vi "ITU_Amplitude(Frequency Domain).vi"(9 "Frequency":dbl=1000.0 format="%#_13g", 10 "Amplitude":dbl=1.0 format="%#_13g") -> (1 "Amplitude_output":dbl)   [LabVIEW 2015]
doc: "Use this VI to calculate ITU-468 filtered amplitude of a signals FFT"
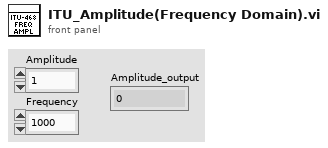
[diagram p1: front panel]
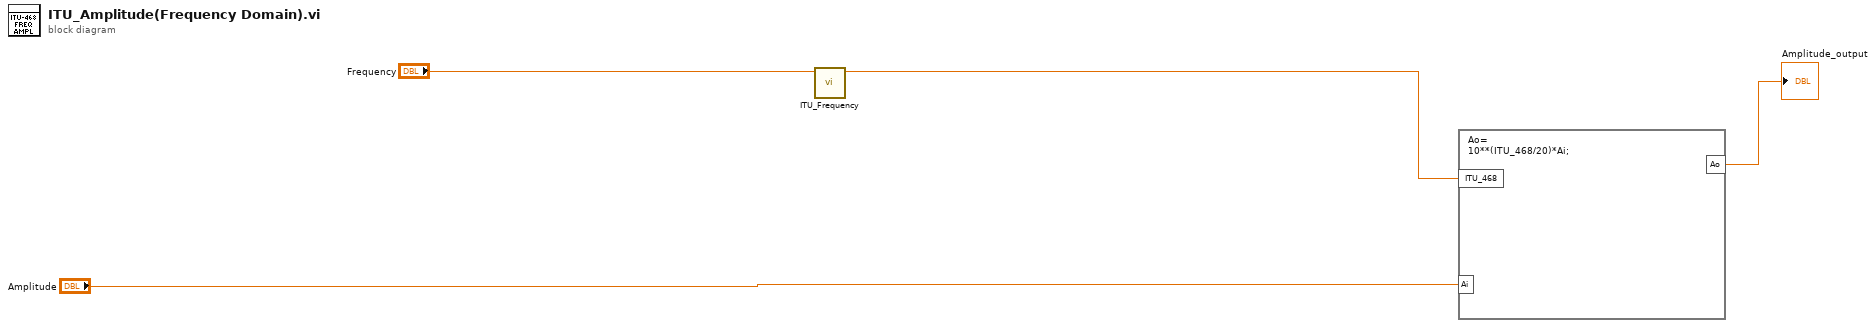
[diagram p0: block diagram]
diagram:
  n1 = call "ITU_Frequency.vi"("Frequency"="Frequency") -> ("ITU_468"=w3:dbl)  [unwired: 10 in]
  n2 = formula code="Ao=\n10**(ITU_468/20)*Ai;"("Ai"="Amplitude", "ITU_468"=w3) -> ("Ao"=→"Amplitude_output":dbl)
